vi "Cam0 Ball Target Loop.vi"(0 "Camera Name":string="cam0") -> ()   [LabVIEW 2023]
uses:
  <vilib>/vision/Image Controls.llb/IMAQ Image.ctl
  Camera Set Up/Event Setup Types.ctl
  <vilib>/Rock Robotics/Network Tables/NT Write Numeric Array.vi
  <vilib>/Utility/config.llb/Write Key (String).vi
  <vilib>/Utility/config.llb/Read Key (String).vi
  <vilib>/Utility/config.llb/NI_LVConfig.lvlib
  <vilib>/vision/NI_Vision_Development_Module.lvlib
panel:
  in  "Main":enum32{"Page 1", "Page 2"}(tab)
  in  "Train Red":bool
  out "Red Distance":dbl[](array[numeric]) caption="Distance" format="%.1f"
  out "Red Angle":dbl[](array[numeric]) caption="Angle" format="%.1f"
  out "Blue Distance":dbl[](array[numeric]) format="%.1f"
  out "Blue Angle":dbl[](array[numeric]) format="%.1f"
  out "Image":T1(plugin-control)
  in  "Settings":bool
  in  "Save":bool
  in  "Tools":bool
  in  "Home":bool
  out "Ball Fps":dbl format="%#.0f"
  in  "Ball Diameter (in)":dbl=10.0
  in  "FOV":dbl=120.0
  in  "Red Color Range":T2={"Hue"={21.620689392089844, 69.62068939208984}, "Sat"={66.41378784179688, 255.0}, "Val"={96.0, 255.0}} caption="Color Range" {"Hue" scale=0.0..255.0 scale format="%#_3g"}
  in  "Blue Color Range":T2={"Hue"={21.620689392089844, 69.62068939208984}, "Sat"={66.41378784179688, 255.0}, "Val"={96.0, 255.0}} caption="Color Range" {"Hue" scale=0.0..255.0 scale format="%#_3g"}
  out "Mask":T1(plugin-control)
  in  "Score Threshold %":dbl=80.0
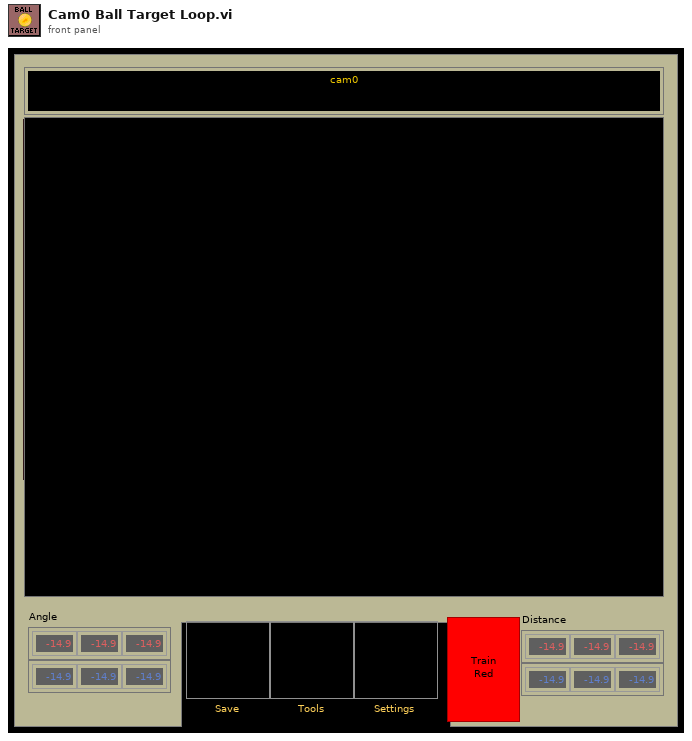
[diagram p1: front panel]
types:
  T1 = typedef "IMAQ Image.ctl" = refnum<image>
  T2 = cluster{"Hue":cluster{dbl, dbl}, "Sat":cluster{dbl, dbl}, "Val":cluster{dbl, dbl}}
  T3 = typedef "Image Type" = u32
  T4 = typedef "Particle Parameters" = i32
  T5 = typedef "Event Setup Types.ctl" = enum16{"Default", "Camera Loop Started", "Save Data", "Open Front Panel", "Exit"}
  T6 = typedef "Target Fields.ctl" = cluster{"diameter points":cluster{"first point":cluster{"x":dbl, "y":dbl}, "projected point":cluster{"x":dbl, "y":dbl}}, "normalized center":cluster{"x":dbl, "y":dbl}, "Overall Score":dbl, "Area Score":dbl, "Moment Score":dbl, "Aspect Score":dbl, "Distance (ft)":dbl, "Upper Goal":bool}
  T7 = typedef "NI_LVConfig.lvlib/Config Data RefNum.ctl" = refnum<k1>
  T8 = cluster{cluster{"Lower":dbl, "Upper":dbl}, cluster{"Lower":dbl, "Upper":dbl}, cluster{"Lower":dbl, "Upper":dbl}}
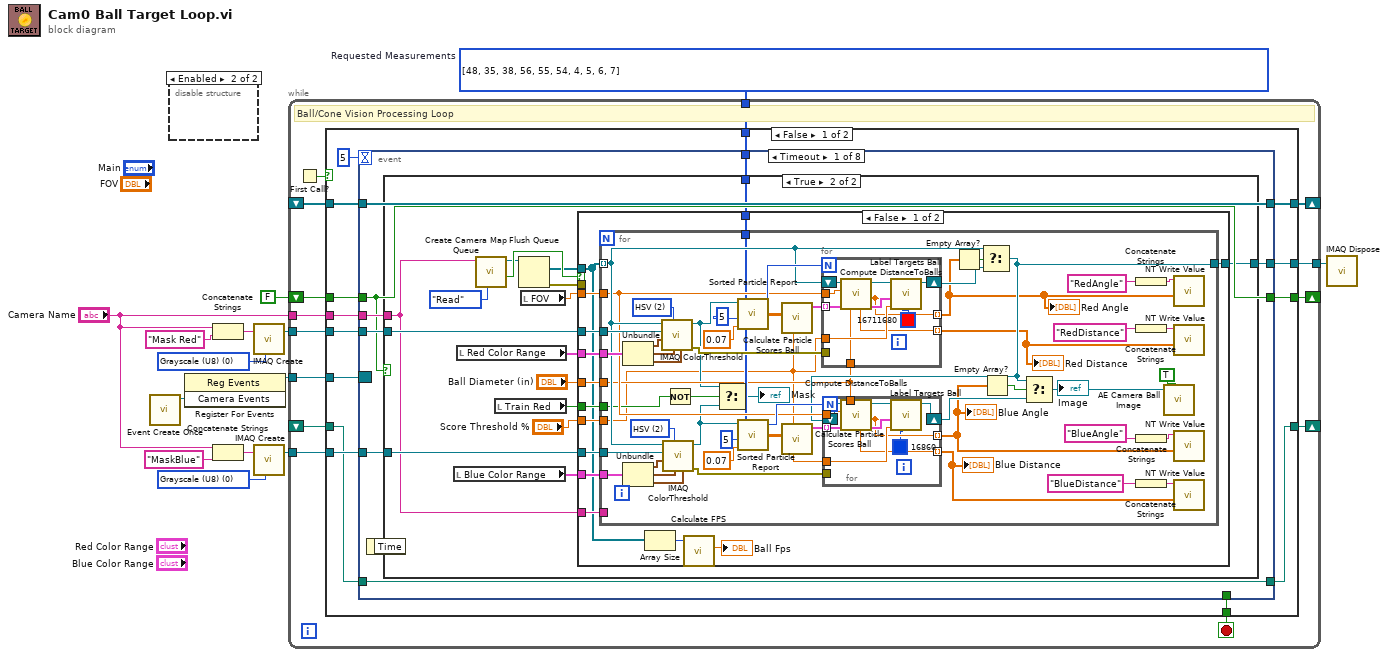
[diagram p0: block diagram]
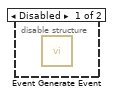
[diagram p2: hidden frame]
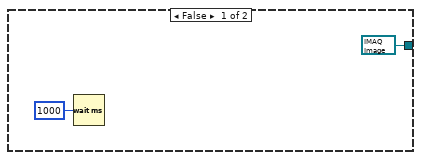
[diagram p3: hidden frame]
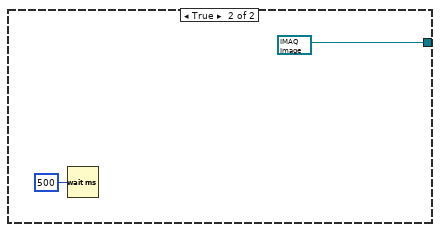
[diagram p4: hidden frame]
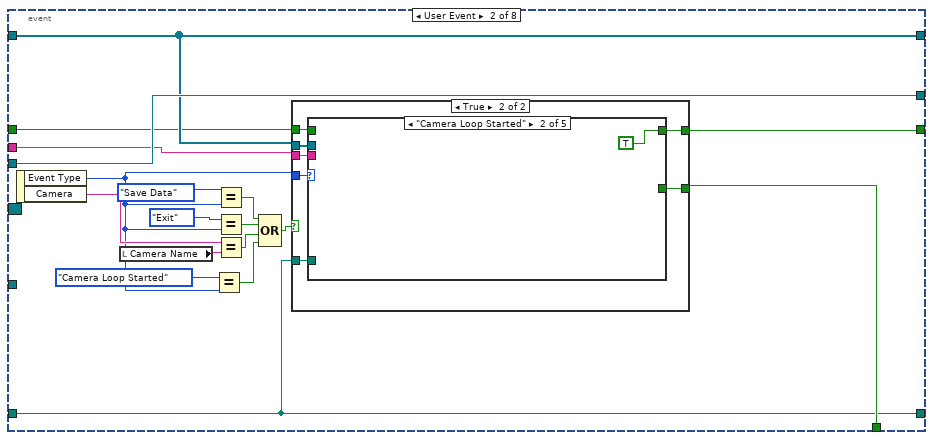
[diagram p5: hidden frame]
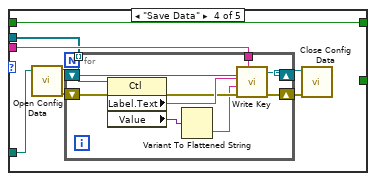
[diagram p9: hidden frame]
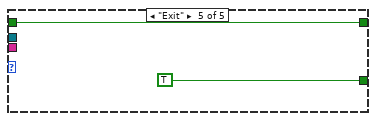
[diagram p10: hidden frame]
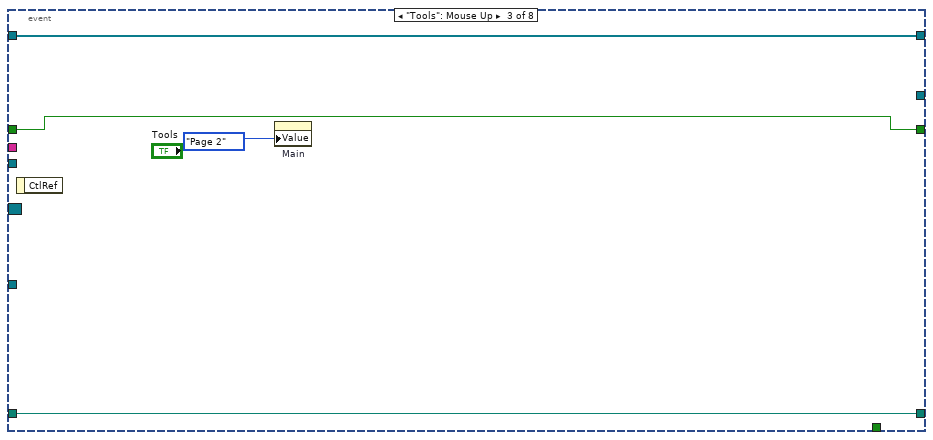
[diagram p11: hidden frame]
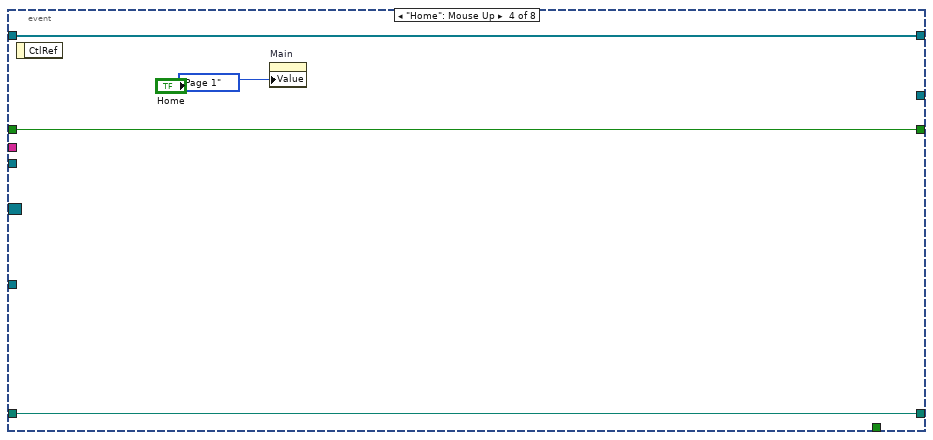
[diagram p12: hidden frame]
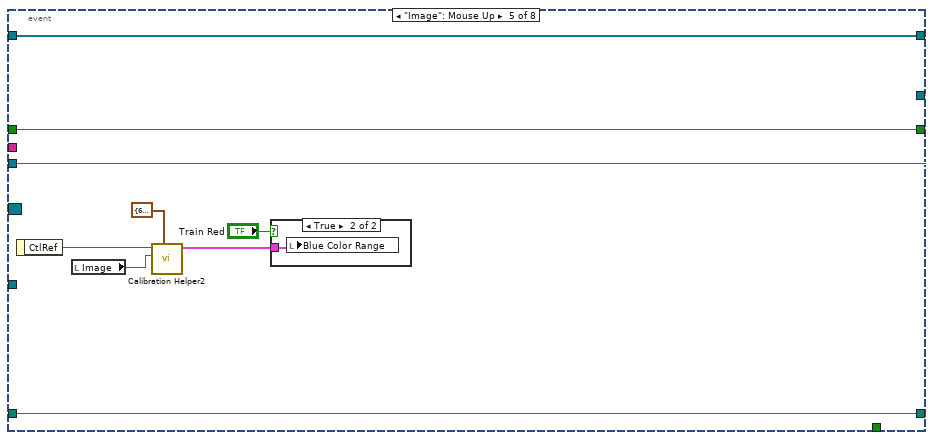
[diagram p13: hidden frame]
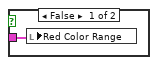
[diagram p14: hidden frame]
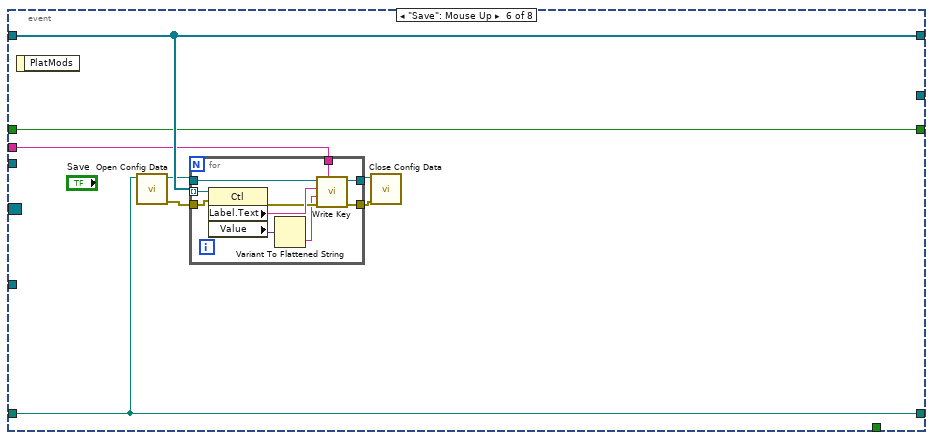
[diagram p15: hidden frame]
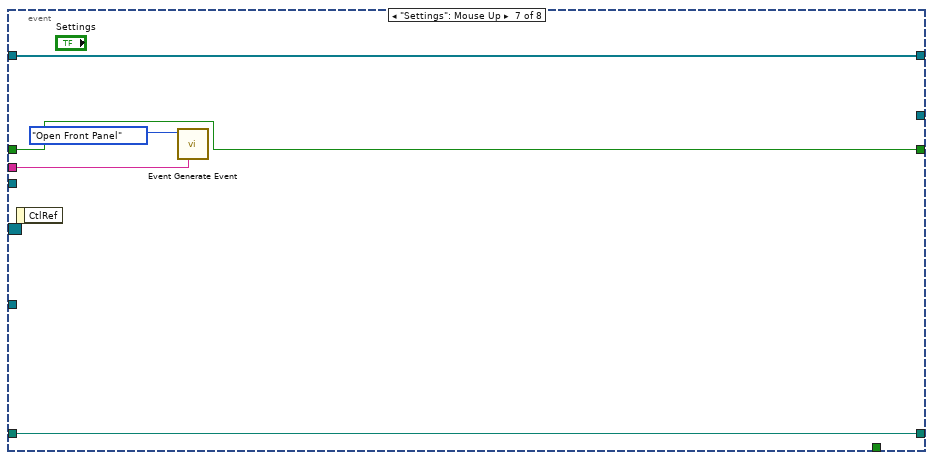
[diagram p16: hidden frame]
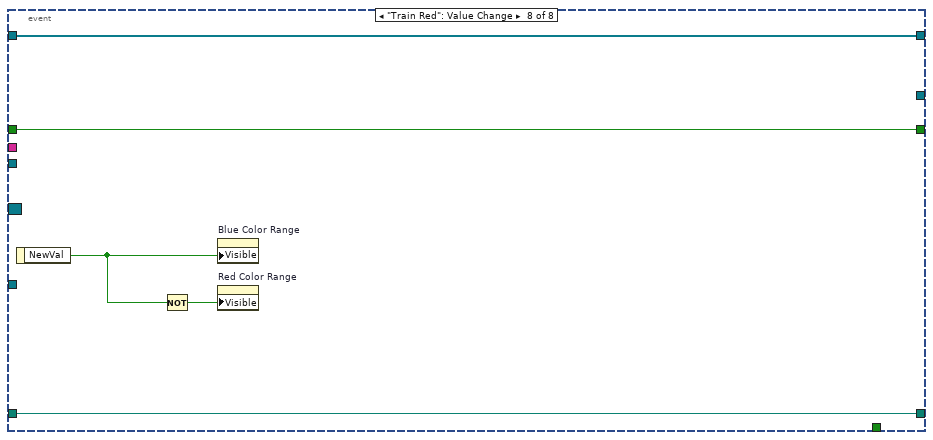
[diagram p17: hidden frame]
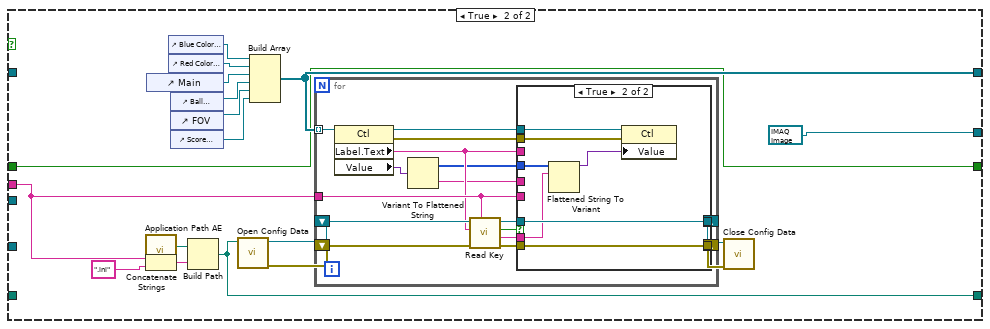
[diagram p18: hidden frame]
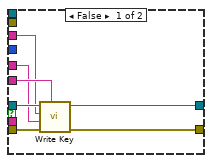
[diagram p19: hidden frame]
diagram:
  w4 = T3 0 items=["Grayscale (U8)", "Grayscale (I16)", "Grayscale (SGL)", "Complex (CSG)", "RGB (U32)", "HSL (U32)", "RGB (U64)", "Grayscale (U16)"] ("Image Type")
  w9 = T4[] [48, 35, 38, 56, 55, 54, 4, 5, 6, 7] items=["Center of Mass X", "Center of Mass Y", "First Pixel X", "First Pixel Y", "Bounding Rect Left", "Bounding Rect Top", "Bounding Rect Right", "Bounding Rect Bottom", "Max Feret Diameter Start X", "Max Feret Diameter Start Y", "Max Feret Diameter End X", "Max Feret Diameter End Y", "Max Horiz. Segment Length Left", "Max Horiz. Segment Length Right", "Max Horiz. Segment Length Row", "-", "Bounding Rect Width", "Bounding Rect Height", "Bounding Rect Diagonal", "Perimeter", "Convex Hull Perimeter", "Holes' Perimeter", "Max Feret Diameter", "Equivalent Ellipse Major Axis", "Equivalent Ellipse Minor Axis", "Equivalent Ellipse Minor Axis (Feret)", "Equivalent Rect Long Side", "Equivalent Rect Short Side", "Equivalent Rect Diagonal", "Equivalent Rect Short Side (Feret)", "Average Horiz. Segment Length", "Average Vert. Segment Length", "Hydraulic Radius", "Waddel Disk Diameter", "-", "Area", "Holes' Area", "Particle & Holes' Area", "Convex Hull Area", "Image Area", "-", "Number of Holes", "Number of Horiz. Segments", "Number of Vert. Segments", "-", "Orientation", "Max Feret Diameter Orientation", "-", "% Area/Image Area", "% Area/(Particle & Holes' Area)", "Ratio of Equivalent Ellipse Axes", "Ratio of Equivalent Rect Sides", "-", "Elongation Factor", "Compactness Factor", "Heywood Circularity Factor", "Type Factor", "-", "Sum X", "Sum Y", "Sum XX", "Sum XY", "Sum YY", "Sum XXX", "Sum XXY", "Sum XYY", "Sum YYY", "-", "Moment of Inertia XX", "Moment of Inertia XY", "Moment of Inertia YY", "Moment of Inertia XXX", "Moment of Inertia XXY", "Moment of Inertia XYY", "Moment of Inertia YYY", "Norm. Moment of Inertia XX", "Norm. Moment of Inertia XY", "Norm. Moment of Inertia YY", "Norm. Moment of Inertia XXX", "Norm. Moment of Inertia XXY", "Norm. Moment of Inertia XYY", "Norm. Moment of Inertia YYY", "Hu Moment 1", "Hu Moment 2", "Hu Moment 3", "Hu Moment 4", "Hu Moment 5", "Hu Moment 6", "Hu Moment 7"]  # Requested Measurements
  w10 = T3 0 items=["Grayscale (U8)", "Grayscale (I16)", "Grayscale (SGL)", "Complex (CSG)", "RGB (U32)", "HSL (U32)", "RGB (U64)", "Grayscale (U16)"] ("Image Type")
  n1 = call "Event Create Once.vi"() -> ("Camera Events"=w12:refnum<user-event>)  [unwired: 10 in, 1 out]
  n2 = disable-structure shown="Enabled" {
    frame Disabled {
      n3 = call "Event Generate Event.vi"() -> ()  [unwired: 12 in]
    }
    frame Enabled {
    }
  }
  n4 = register-events(w12) -> (reference out=w11:refnum<event-registration>)  [unwired: 2 in, 1 out]
  n5 = Concatenate Strings("Camera Name", "Mask Red" ("string")) -> (w8:string)
  n6 = Concatenate Strings("Camera Name", "MaskBlue" ("string")) -> (w5:string)
  n7 = call "IMAQ Create"("Image Name"=w8, "Image Type"=w10) -> ("New Image"=w14:T1)  [unwired: 2 in, 2 out]
  n8 = call "IMAQ Create"("Image Name"=w5, "Image Type"=w4) -> ("New Image"=w3:T1)  [unwired: 2 in, 2 out]
  n9 = while {
    tunnel: w14 -> [w28]
    tunnel: w9 -> [w27]
    tunnel: [w26] -> w13
    tunnel: w11 -> [w25]
    tunnel: "Camera Name" -> [w23]
    shift-right: [w21] -> _
    shift-left: _ -> [w20]
    shift-right: [w19] -> _
    shift-left: _ -> [w18]
    tunnel: w3 -> [w17]
    shift-right: [w15] -> _
    shift-left: FALSE -> [w16]
    stop <- w24 stop-if-true
    # "Ball/Cone Vision Processing Loop"
    n10 = First Call?() -> (First Call?: T/F=w22:bool)
    n11 = case shown="False" w22 {
      tunnel: w28 -> [w42 _]
      tunnel: w27 -> [w41 _]
      tunnel: [w40 T1 refnum ("New Image")] -> w26
      tunnel: w25 -> [w39 _]
      tunnel: [w38 _] -> w24
      tunnel: w23 -> [w37 w267]
      tunnel: [w35 w262] -> w21
      tunnel: w20 -> [w36 _]
      tunnel: [w34 w266] -> w19
      tunnel: w18 -> [w31 _]
      tunnel: w17 -> [w33 _]
      tunnel: w16 -> [w30 w256]
      tunnel: [w29 w256] -> w15
      frame False {
        n12 = event shown="[0] Timeout" {
          selector: w39 -> [_ _ _ _ _ _ _ _]
          dyn-events: _ -> [_ _ _ _ _ _ _ _]
          timeout: 5 -> [_ _ _ _ _ _ _ _]
          tunnel: w42 -> [w48 w177 _ _ w223 _ _ _]
          tunnel: w41 -> [w50 _ _ _ _ _ _ _]
          tunnel: [w49 w177 _ _ w223 _ _ _] -> w40
          tunnel: [_ w176 _ _ _ _ _ _] -> w38
          tunnel: w37 -> [w44 w175 _ _ _ w231 w247 _]
          tunnel: w36 -> [w47 w173 w212 w216 w221 w234 w250 w255]
          tunnel: [w47 w173 w212 w216 w221 w234 w250 w255] -> w35
          tunnel: w31 -> [w46 w174 w211 w215 w220 w235 w249 w254]
          tunnel: [w46 w174 w211 w215 w220 w235 w249 w254] -> w34
          tunnel: w33 -> [w45 _ _ _ _ _ _ _]
          tunnel: w30 -> [w43 w164 w209 w213 w217 w228 w246 w251]
          tunnel: [w43 w163 w209 w213 w217 w228 w246 w251] -> w29
          event Timeout {
            n13 = event-data() -> ()  [unwired: 1 in, 1 out]
            n14 = case shown="True" w43 {
              tunnel: w50 -> [_ w68]
              tunnel: [T1 refnum ("Image") w67] -> w49
              tunnel: w48 -> [_ w66]
              tunnel: w45 -> [_ w61]
              tunnel: w44 -> [_ w53]
              frame False {
                n15 = Wait (ms)(milliseconds to wait=u32 1000) -> ()  [unwired: 1 out]
              }
              frame True {
                n16 = local read "Blue Color Range"() -> (w60:T2)
                n17 = local read "Red Color Range"() -> (w62:T2)
                n18 = call "Create Camera Map Queue.vi"("Action"=enum16{"Read", "Write"}."Read", "Camera"=w53) -> ("key not found?"=w64:bool, "value"=w56:refnum<queue>)  [unwired: 8 in]
                n19 = local read "Train Red"() -> (w58:bool)
                n20 = Flush Queue(queue=w56) -> (remaining elements=w55:T1[], error out=w54:errorcluster)  [unwired: 1 in, 1 out]
                n21 = local read "FOV"() -> (w63:dbl)
                n22 = case shown="False" w64 {
                  tunnel: w68 -> [w82 _]
                  tunnel: [w81 T1 refnum ("Image")] -> w67
                  tunnel: w66 -> [w80 _]
                  tunnel: w63 -> [w79 _]
                  tunnel: w62 -> [w78 _]
                  tunnel: w61 -> [w77 _]
                  tunnel: w60 -> [w76 _]
                  tunnel: w53 -> [w75 _]
                  tunnel: "Ball Diameter (in)" -> [w74 _]
                  tunnel: w58 -> [w73 _]
                  tunnel: "Score Threshold %" -> [w72 _]
                  tunnel: w55 -> [w69 _]
                  tunnel: w54 -> [_ _]
                  frame False {
                    n23 = for {
                      tunnel: w80 -> [w130]
                      tunnel: w82 -> [w106]
                      tunnel: w69 -> [w109] mode=indexing
                      tunnel: [w104] -> w81
                      tunnel: w79 -> [w107]
                      tunnel: w78 -> [w125]
                      tunnel: w77 -> [w108]
                      tunnel: w76 -> [w105]
                      tunnel: w75 -> [_]
                      tunnel: w74 -> [w91]
                      tunnel: w73 -> [w90]
                      tunnel: w72 -> [w85]
                      w114 = u16 2 items=["RGB", "HSL", "HSV", "HSI"] ("Color Mode")
                      w131 = u16 2 items=["RGB", "HSL", "HSV", "HSI"] ("Color Mode")
                      n24 = Unbundle(w125) -> ("Hue"=w124:cluster{dbl, dbl}, "Sat"=w123:cluster{dbl, dbl}, "Val"=w122:cluster{dbl, dbl})
                      n25 = Unbundle(w105) -> ("Hue"=w119:cluster{dbl, dbl}, "Sat"=w120:cluster{dbl, dbl}, "Val"=w121:cluster{dbl, dbl})
                      n26 = call "IMAQ ColorThreshold"("Blue or Luma or Val or Inten Range"=w122, "Green or Sat Range"=w123, "Color Mode"=w131, "Red or Hue Range"=w124, "Image Dst"=w130, "Image Src"=w109) -> ("error out"=w129:errorcluster, "Image Dst Out"=w87:T1)  [unwired: 4 in]
                      n27 = call "IMAQ ColorThreshold"("Blue or Luma or Val or Inten Range"=w121, "Green or Sat Range"=w120, "Color Mode"=w114, "Red or Hue Range"=w119, "Image Dst"=w108, "Image Src"=w109) -> ("error out"=w115:errorcluster, "Image Dst Out"=w88:T1)  [unwired: 4 in]
                      n28 = Not(x=w90) -> (.not. x?=w86:bool)
                      n29 = Select(t=w87, s=w86, f=w88) -> (s? t:f=→"Mask":T1)
                      n30 = call "Sorted Particle Report.vi"("Min Area Size %"=0.07 ("Size Limit %"), "Particle Count Limit"=5 ("Particle Count LImit"), "Pixel Measurements"=w106, "Image in"=w87) -> ("Sorted Data"=w134:dbl[][], "Particles"=w128:i32)  [unwired: 1 out]
                      n31 = call "Sorted Particle Report.vi"("Min Area Size %"=0.07 ("Size Limit %"), "Particle Count Limit"=5 ("Particle Count LImit"), "Pixel Measurements"=w106, "Image in"=w88) -> ("Sorted Data"=w111:dbl[][], "Particles"=w116:i32)  [unwired: 1 out]
                      n32 = call "Calculate Particle Scores Ball.vi"("Limit"=w85, "Sorted Data"=w134) -> ("Scores"=w133:T6[])  [unwired: 9 in]
                      n33 = call "Calculate Particle Scores Ball.vi"("Limit"=w85, "Sorted Data"=w111) -> ("Scores"=w112:T6[])  [unwired: 9 in]
                      n34 = for {
                        N: w128 -> [_]
                        tunnel: w133 -> [w155] mode=indexing
                        shift-right: [w157] -> w127
                        shift-left: w109 -> [w153]
                        tunnel: w85 -> [w156]
                        tunnel: [w150] -> w93 mode=indexing
                        tunnel: w129 -> [_]
                        tunnel: w107 -> [w151]
                        tunnel: [w149] -> w92 mode=indexing
                        tunnel: w91 -> [w147]
                        n35 = call "Compute DistanceToBalls.vi"("Target Width (in)"=w147, "results"=w155, "FOV"=w151, "Image Src"=w153) -> ("results out"=w152:T6, "Off Angle"=w150:dbl, "Image Dst Out"=w154:T1, "Distance"=w149:dbl)  [unwired: 3 in, 1 out]
                        n36 = call "Label Targets Ball.vi"("Color"=u32 16711680, "Score Threshold"=w156, "results"=w152, "Angle"=w150, "Image in"=w154) -> ("Image out"=w157:T1)  [unwired: 6 in]
                      }
                      "Red Angle" <- w93
                      "Red Distance" <- w92
                      n37 = Empty Array?(array=w93) -> (empty?=w126:bool)
                      n38 = Select(t=w109, s=w126, f=w127) -> (s? t:f=w104:T1)
                      n39 = for {
                        N: w116 -> [_]
                        tunnel: w112 -> [w144] mode=indexing
                        shift-right: [w146] -> w117
                        shift-left: w104 -> [w142]
                        tunnel: w85 -> [w145]
                        tunnel: [w139] -> w103 mode=indexing
                        tunnel: w115 -> [_]
                        tunnel: w107 -> [w140]
                        tunnel: [w138] -> w102 mode=indexing
                        tunnel: w91 -> [w136]
                        n40 = call "Compute DistanceToBalls.vi"("Target Width (in)"=w136, "results"=w144, "FOV"=w140, "Image Src"=w142) -> ("results out"=w141:T6, "Off Angle"=w139:dbl, "Image Dst Out"=w143:T1, "Distance"=w138:dbl)  [unwired: 3 in, 1 out]
                        n41 = call "Label Targets Ball.vi"("Color"=u32 16860, "Score Threshold"=w145, "results"=w141, "Angle"=w139, "Image in"=w143) -> ("Image out"=w146:T1)  [unwired: 6 in]
                      }
                      "Blue Angle" <- w103
                      "Blue Distance" <- w102
                      n42 = Empty Array?(array=w103) -> (empty?=w118:bool)
                      n43 = Select(t=w104, s=w118, f=w117) -> (s? t:f=w84:T1)
                      "Image" <- w84
                      n44 = Concatenate Strings("RedAngle" ("Name")) -> (w94:string)
                      n45 = Concatenate Strings("RedDistance" ("Name")) -> (w95:string)
                      n46 = Concatenate Strings("BlueAngle" ("Name")) -> (w98:string)
                      n47 = Concatenate Strings("BlueDistance" ("Name")) -> (w100:string)
                      n48 = call "AE Camera Ball Image.vi"("Update"=TRUE, "Ball Image in"=w84) -> ()  [unwired: 9 in, 1 out]
                      n49 = call-poly <vilib>:"NT Write Value.vi"("value"=w93, "name"=w94) -> ()  [unwired: 9 in, 1 out]
                      n50 = call-poly <vilib>:"NT Write Value.vi"("value"=w92, "name"=w95) -> ()  [unwired: 9 in, 1 out]
                      n51 = call-poly <vilib>:"NT Write Value.vi"("value"=w103, "name"=w98) -> ()  [unwired: 9 in, 1 out]
                      n52 = call-poly <vilib>:"NT Write Value.vi"("value"=w102, "name"=w100) -> ()  [unwired: 9 in, 1 out]
                    }
                    n53 = Array Size(array=w69) -> (size(s)=w71:i32)
                    n54 = call "Calculate FPS.vi"("Frames Processed"=w71) -> ("Fps"=→"Ball Fps":dbl)  [unwired: 10 in]
                  }
                  frame True {
                    n55 = Wait (ms)(milliseconds to wait=u32 500) -> ()  [unwired: 1 out]
                  }
                }
              }
            }
          }
          event User Event {
            n56 = event-data() -> ("Event Type"=w162:T5, "Camera"=w167:string)  [unwired: 1 in]
            n57 = local read "Camera Name"() -> (w168:string)
            n58 = Equal?(x=Event_Setup_Types."Camera Loop Started", y=w162) -> (x = y?=w160:bool)
            n59 = Equal?(x=Event_Setup_Types."Save Data", y=w162) -> (x = y?=w169:bool)
            n60 = Equal?(x=Event_Setup_Types."Exit", y=w162) -> (x = y?=w171:bool)
            n61 = Equal?(x=w167, y=w168) -> (x = y?=w166:bool)
            n62 = Compound Arithmetic op=OR(w169, w171, w166, w160) -> (w165:bool)
            n63 = case shown="True" w165 {
              tunnel: w162 -> [_ w185]
              tunnel: [_ w184] -> w176
              tunnel: w175 -> [_ w183]
              tunnel: w174 -> [_ w182]
              tunnel: w173 -> [_ w181]
              tunnel: w164 -> [w178 w180]
              tunnel: [w178 w179] -> w163
              frame False {
              }
              frame True {
                n64 = case shown="\"Camera Loop Started\"" w185 {
                  tunnel: [_ _ _ _ TRUE] -> w184
                  tunnel: w183 -> [_ _ _ w192 _]
                  tunnel: w182 -> [_ _ _ w191 _]
                  tunnel: w181 -> [_ _ _ w190 _]
                  tunnel: w180 -> [w186 _ w188 w189 w207]
                  tunnel: [w186 TRUE w188 w189 w207] -> w179
                  frame "Default" {
                  }
                  frame "Camera Loop Started" {
                  }
                  frame "Open Front Panel" {
                  }
                  frame "Save Data" {
                    n65 = call <vilib>:"Open Config Data.vi"("configuration file path"=w191) -> ("error out"=w193:errorcluster, "refnum"=w196:T7)  [unwired: 8 in, 1 out]
                    n66 = for {
                      tunnel: w192 -> [w202]
                      tunnel: w190 -> [w201] mode=indexing
                      shift-right: [w205] -> w195
                      shift-left: w196 -> [w206]
                      shift-right: [w204] -> w194
                      shift-left: w193 -> [w203]
                      n67 = property class="Ctl"(reference=w201, error in=w203) -> (error out=w198:errorcluster, "Label.Text"=w200:string, "Value"=w199:variant)  [unwired: 1 out]
                      n68 = Variant To Flattened String(Variant=w199) -> (data string=w197:string)  [unwired: 1 out]
                      n69 = call-poly <vilib>:"Write Key.vi"("section"=w202, "error in (no error)"=w198, "value"=w197, "key"=w200, "refnum"=w206) -> ("error out"=w204:errorcluster, "refnum out"=w205:T7)  [unwired: 4 in, 1 out]
                    }
                    n70 = call <vilib>:"Close Config Data.vi"("error in (no error)"=w194, "refnum"=w195) -> ()  [unwired: 8 in, 2 out]
                  }
                  frame "Exit" {
                  }
                }
              }
            }
          }
          event "Tools": Mouse Up {
            n71 = event-data() -> ()  [unwired: 1 in, 1 out]
            n72 = property on="Main" class="TabCtl (strict)"("Value"=enum32{"Page 1", "Page 2"}."Page 2" ("Main")) -> ()  [unwired: 2 in, 2 out]
          }
          event "Home": Mouse Up {
            n73 = event-data() -> ()  [unwired: 1 in, 1 out]
            n74 = property on="Main" class="TabCtl (strict)"("Value"=enum32{"Page 1", "Page 2"}."Page 1" ("Main")) -> ()  [unwired: 2 in, 2 out]
          }
          event "Image": Mouse Up {
            n75 = event-data() -> ("CtlRef"=w224:refnum<vi>)  [unwired: 1 in]
            n76 = local read "Image"() -> (w222:T1)
            n77 = call "Calibration Helper2.vi"("Std Devs"=cluster{"H":dbl, "S":dbl, "V":dbl} {"H"=6.0, "S"=6.0, "V"=6.0} ("Std Devs Ball"), "Image"=w222, "Image Ctl Refnum"=w224) -> ("output color"=w218:T8)  [unwired: 7 in, 1 out]
            n78 = case shown="True" "Train Red" {
              tunnel: w218 -> [w226 w227]
              frame False {
                n79 = local write "Red Color Range"(w226) -> ()
              }
              frame True {
                n80 = local write "Blue Color Range"(w227) -> ()
              }
            }
          }
          event "Save": Mouse Up {
            n81 = event-data() -> ()  [unwired: 1 in, 1 out]
            n82 = call <vilib>:"Open Config Data.vi"("configuration file path"=w235) -> ("error out"=w232:errorcluster, "refnum"=w233:T7)  [unwired: 8 in, 1 out]
            n83 = for {
              tunnel: w234 -> [w245] mode=indexing
              tunnel: w233 -> [w244]
              tunnel: w232 -> [w243]
              tunnel: w231 -> [w239]
              tunnel: [w237] -> w230
              tunnel: [w236] -> w229
              n84 = property class="Ctl"(reference=w245, error in=w243) -> (error out=w240:errorcluster, "Label.Text"=w242:string, "Value"=w241:variant)  [unwired: 1 out]
              n85 = Variant To Flattened String(Variant=w241) -> (data string=w238:string)  [unwired: 1 out]
              n86 = call-poly <vilib>:"Write Key.vi"("section"=w239, "error in (no error)"=w240, "value"=w238, "key"=w242, "refnum"=w244) -> ("error out"=w237:errorcluster, "refnum out"=w236:T7)  [unwired: 4 in, 1 out]
            }
            n87 = call <vilib>:"Close Config Data.vi"("error in (no error)"=w230, "refnum"=w229) -> ()  [unwired: 8 in, 2 out]
          }
          event "Settings": Mouse Up {
            n88 = event-data() -> ()  [unwired: 1 in, 1 out]
            n89 = call "Event Generate Event.vi"("Camera Name"=w247, "Event Type"=Event_Setup_Types."Open Front Panel") -> ()  [unwired: 10 in]
          }
          event "Train Red": Value Change {
            n90 = event-data() -> ("NewVal"=w253:bool)  [unwired: 1 in]
            n91 = Not(x=w253) -> (.not. x?=w252:bool)
            n92 = property on="Blue Color Range" class="Clust (strict)"("Visible"=w253) -> ()  [unwired: 2 in, 2 out]
            n93 = property on="Red Color Range" class="Clust (strict)"("Visible"=w252) -> ()  [unwired: 2 in, 2 out]
          }
        }
      }
      frame True {
        n94 = call "Application Path AE.vi"() -> ("Application Path out"=w264:path)  [unwired: 11 in]
        n95 = Concatenate Strings(w267, ".ini" ("name or relative path")) -> (w272:string)
        n96 = control-ref of="Main"() -> (w261:refnum<vi>)
        n97 = control-ref of="Blue Color Range"() -> (w260:refnum<vi>)
        n98 = control-ref of="Red Color Range"() -> (w263:refnum<vi>)
        n99 = control-ref of="Ball Diameter (in)"() -> (w259:refnum<vi>)
        n100 = control-ref of="FOV"() -> (w258:refnum<vi>)
        n101 = control-ref of="Score Threshold %"() -> (w257:refnum<vi>)
        n102 = Build Path(base path=w264, name or relative path=w272) -> (appended path=w266:path)
        n103 = call <vilib>:"Open Config Data.vi"("configuration file path"=w266) -> ("error out"=w265:errorcluster, "refnum"=w271:T7)  [unwired: 8 in, 1 out]
        n104 = Build Array(w260, w263, w261, w259, w258, w257) -> (w262:refnum<vi>[])
        n105 = for {
          tunnel: w267 -> [w286]
          tunnel: w262 -> [w276] mode=indexing
          shift-right: [w288] -> w270
          shift-left: w271 -> [w289]
          shift-right: [w287] -> w269
          shift-left: w265 -> [w285]
          n106 = property class="Ctl"(reference=w276) -> (reference out=w282:refnum<vi>, error out=w281:errorcluster, "Label.Text"=w279:string, "Value"=w275:variant)  [unwired: 1 in]
          n107 = Variant To Flattened String(Variant=w275) -> (data string=w277:string, 1:w274:i16[])
          n108 = call-poly <vilib>:"Read Key.vi"("section"=w286, "error in (no error)"=w285, "key"=w279, "refnum"=w289) -> ("error out"=w278:errorcluster, "value"=w283:string, "found?"=w284:bool, "refnum out"=w280:T7)  [unwired: 4 in]
          n109 = case shown="True" w284 {
            tunnel: w283 -> [_ w298]
            tunnel: w282 -> [_ w303]
            tunnel: w281 -> [_ w302]
            tunnel: w280 -> [w296 w301]
            tunnel: w286 -> [w295 _]
            tunnel: w279 -> [w294 _]
            tunnel: [w293 w301] -> w288
            tunnel: w278 -> [w292 w300]
            tunnel: [w291 w300] -> w287
            tunnel: w277 -> [w290 _]
            tunnel: w274 -> [_ w297]
            frame False {
              n110 = call-poly <vilib>:"Write Key.vi"("section"=w295, "error in (no error)"=w292, "value"=w290, "key"=w294, "refnum"=w296) -> ("error out"=w291:errorcluster, "refnum out"=w293:T7)  [unwired: 4 in, 1 out]
            }
            frame True {
              n111 = Flattened String To Variant(6:w298, 7:w297) -> (3:w299:variant)  [unwired: 1 in, 1 out]
              n112 = property class="Ctl"(reference=w303, error in=w302, "Value"=w299) -> ()  [unwired: 2 out]
            }
          }
        }
        n113 = call <vilib>:"Close Config Data.vi"("error in (no error)"=w269, "refnum"=w270) -> ()  [unwired: 8 in, 2 out]
      }
    }
  }
  n114 = call "IMAQ Dispose"("Image"=w13) -> ()  [unwired: 5 in, 1 out]
